vi "ldr.vi"() -> ()   [LabVIEW 2017]
panel:
  out "Low Lighing":bool
  out "LDR Output (V)":dbl
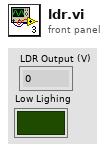
[diagram p1: front panel]
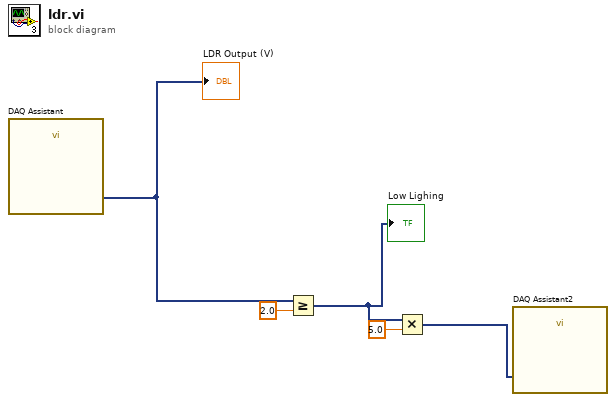
[diagram p0: block diagram]
diagram:
  n1 = call "DAQ Assistant"() -> ("data"=w5:dynamicdata)  [unwired: 16 in, 3 out]
  "LDR Output (V)" <- w5
  n2 = Greater Or Equal?(x=w5, y=2.0) -> (x >= y?=w2:dynamicdata)
  "Low Lighing" <- w2
  n3 = Multiply(x=w2, y=5.0) -> (x*y=w1:dynamicdata)
  n4 = call "DAQ Assistant2"("data"=w1) -> ()  [unwired: 16 in, 3 out]
